vi "Yokogawa - single module.vi"(10 "Module to save":i32, 11 "Electrical Data Out in":T1) -> (3 "Electrical Data Out out":T1)   [LabVIEW 2013]
uses:
  electrical2.ctl
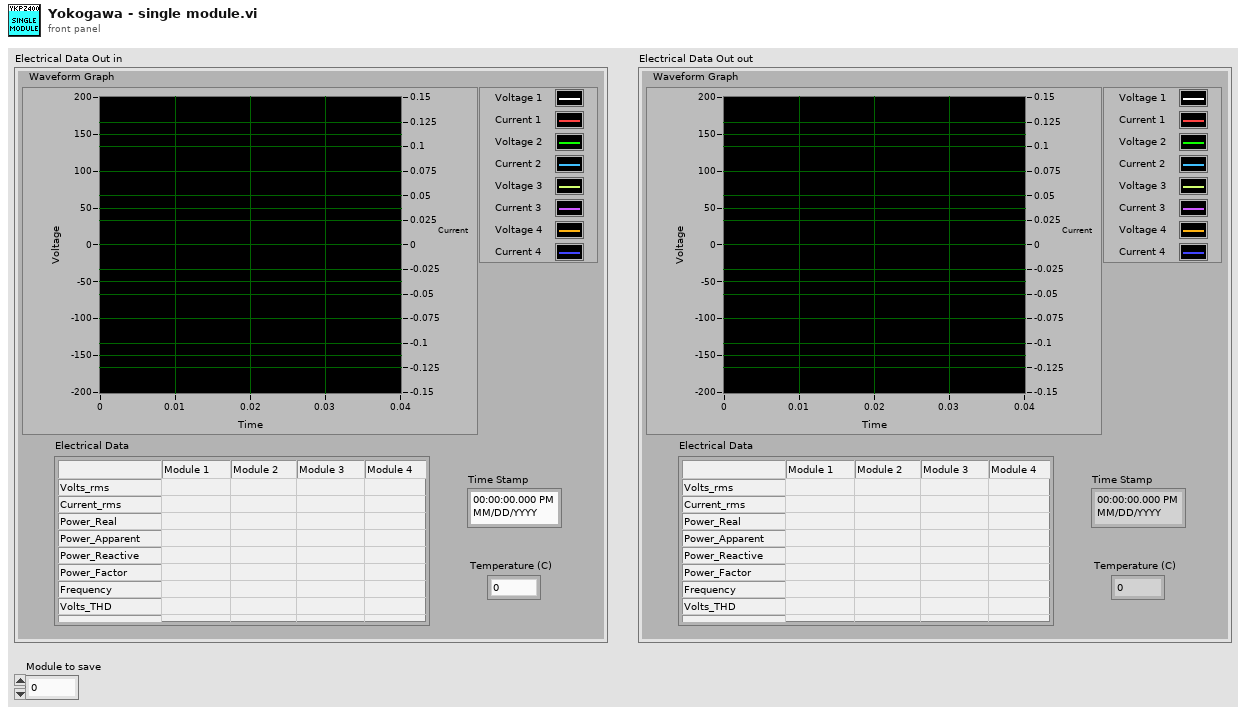
[diagram p1: front panel]
types:
  T1 = typedef "electrical2.ctl" = cluster{"Time Stamp":timestamp, "Temperature (C)":dbl, "Electrical Data":string[][], "Waveform Graph":waveform(dbl)[]}
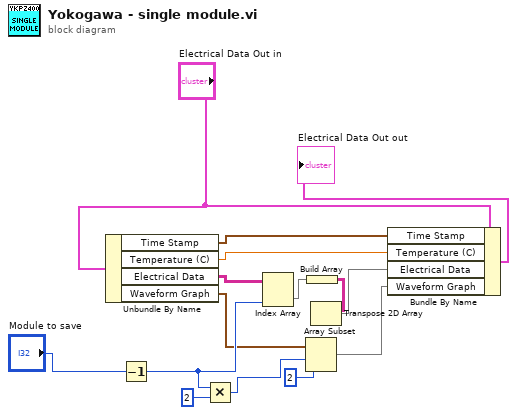
[diagram p0: block diagram]
diagram:
  n1 = Unbundle By Name("Electrical Data Out in") -> ("Time Stamp"=w5:timestamp, "Temperature (C)"=w6:dbl, "Electrical Data"=w1:string[][], "Waveform Graph"=w2:waveform(dbl)[])
  n2 = Decrement(x="Module to save") -> (x-1=w13:i32)
  n3 = Multiply(x=w13, y=2) -> (x*y=w15:i32)
  n4 = Index Array(array=w1, index (col)=w13) -> (element=w7:string[])  [unwired: 1 in]
  n5 = Array Subset(array=w2, index=w15, length=2) -> (w8:waveform(dbl)[])
  n6 = Build Array(w7) -> (w10:string[][])
  n7 = Transpose 2D Array(2D array=w10) -> (transposed array=w11:string[][])
  n8 = Bundle By Name(cluster="Electrical Data Out in", "Time Stamp"=w5, "Temperature (C)"=w6, "Electrical Data"=w11, "Waveform Graph"=w8) -> (→"Electrical Data Out out":T1)
